vi "Close.vi"(8 "error in":errorcluster, 11 "Cycler in":refnum<class "Cycler.lvclass">) -> (0 "error out":errorcluster, 3 "Cycler out":refnum<class "Cycler.lvclass">)   [LabVIEW 2023, in "Cycler.lvclass"]
uses:
  Cycler.lvclass
  Cycler.lvclass/Cycler.ctl
  Low Level Capabilities/OnOff/OnOff.lvclass
  Low Level Capabilities/Output Enable/Output Enable.lvclass
  Low Level Capabilities/Control Mode/Control Mode.lvclass
  Low Level Capabilities/Current/Current Actual Value/Current Actual Value.lvclass
  Low Level Capabilities/Current/Current Gradient/Current Gradient.lvclass
  Low Level Capabilities/Current/Current Limit/Current Limit.lvclass
  Low Level Capabilities/Current/Current Setpoint/Current Setpoint.lvclass
  Low Level Capabilities/Power/Power Actual Value/Power Actual Value.lvclass
  Low Level Capabilities/Power/Power Gradient/Power Gradient.lvclass
  Low Level Capabilities/Power/Power Limit/Power Limit.lvclass
  Low Level Capabilities/Power/Power Setpoint/Power Setpoint.lvclass
  Low Level Capabilities/Voltage/Voltage Actual Value/Voltage Actual Value.lvclass
  Low Level Capabilities/Voltage/Voltage Gradient/Voltage Gradient.lvclass
  Low Level Capabilities/Voltage/Voltage Limit/Voltage Limit.lvclass
  Low Level Capabilities/Voltage/Voltage Setpoint/Voltage Setpoint.lvclass
  Low Level Capabilities/Error/Error.lvclass
  Low Level Capabilities/Error Channels/Error Channels.lvclass
  Low Level Capabilities/Iso Measurement/Iso Measurement.lvclass
  Low Level Capabilities/Parallel Mode/Parallel Mode.lvclass
  Low Level Capabilities/Parameter Set/Parameter Set.lvclass
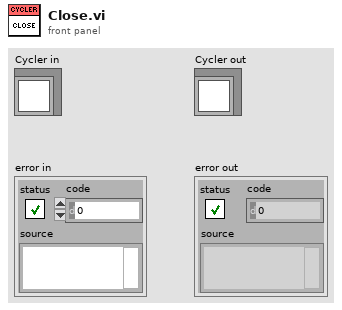
[diagram p1: front panel]
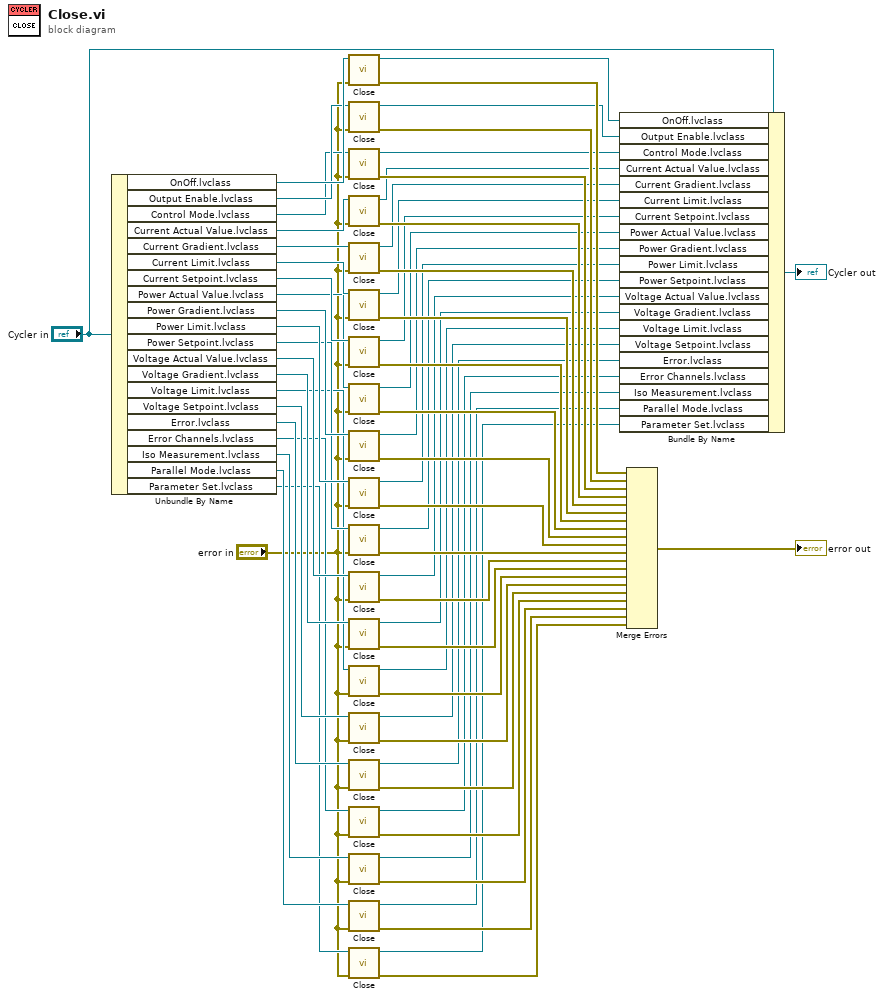
[diagram p0: block diagram]
diagram:
  n1 = Unbundle By Name("Cycler in") -> ("OnOff.lvclass"=w62:refnum<class "OnOff.lvclass">, "Output Enable.lvclass"=w59:refnum<class "Output Enable.lvclass">, "Control Mode.lvclass"=w56:refnum<class "Control Mode.lvclass">, "Current Actual Value.lvclass"=w53:refnum<class "Current Actual Value.lvclass">, "Current Gradient.lvclass"=w50:refnum<class "Current Gradient.lvclass">, "Current Limit.lvclass"=w47:refnum<class "Current Limit.lvclass">, "Current Setpoint.lvclass"=w44:refnum<class "Current Setpoint.lvclass">, "Power Actual Value.lvclass"=w41:refnum<class "Power Actual Value.lvclass">, "Power Gradient.lvclass"=w38:refnum<class "Power Gradient.lvclass">, "Power Limit.lvclass"=w35:refnum<class "Power Limit.lvclass">, "Power Setpoint.lvclass"=w32:refnum<class "Power Setpoint.lvclass">, "Voltage Actual Value.lvclass"=w29:refnum<class "Voltage Actual Value.lvclass">, "Voltage Gradient.lvclass"=w26:refnum<class "Voltage Gradient.lvclass">, "Voltage Limit.lvclass"=w23:refnum<class "Voltage Limit.lvclass">, "Voltage Setpoint.lvclass"=w20:refnum<class "Voltage Setpoint.lvclass">, "Error.lvclass"=w17:refnum<class "Error.lvclass">, "Error Channels.lvclass"=w14:refnum<class "Error Channels.lvclass">, "Iso Measurement.lvclass"=w11:refnum<class "Iso Measurement.lvclass">, "Parallel Mode.lvclass"=w6:refnum<class "Parallel Mode.lvclass">, "Parameter Set.lvclass"=w5:refnum<class "Parameter Set.lvclass">)
  n2 = call-dynamic "Close.vi"("error in"="error in", "OnOff in"=w62) -> ("error out"=w60:errorcluster, "OnOff out"=w61:refnum<class "OnOff.lvclass">)  [unwired: 8 in]
  n3 = call-dynamic "Close.vi"("error in"="error in", "Output Enable in"=w59) -> ("error out"=w57:errorcluster, "Output Enable out"=w58:refnum<class "Output Enable.lvclass">)  [unwired: 8 in]
  n4 = call-dynamic "Close.vi"("error in"="error in", "Control Mode in"=w56) -> ("error out"=w55:errorcluster, "Control Mode out"=w54:refnum<class "Control Mode.lvclass">)  [unwired: 8 in]
  n5 = call-dynamic "Close.vi"("error in"="error in", "Current Actual Value in"=w53) -> ("error out"=w52:errorcluster, "Current Actual Value out"=w51:refnum<class "Current Actual Value.lvclass">)  [unwired: 8 in]
  n6 = call-dynamic "Close.vi"("error in"="error in", "Current Gradient in"=w50) -> ("error out"=w49:errorcluster, "Current Gradient out"=w48:refnum<class "Current Gradient.lvclass">)  [unwired: 8 in]
  n7 = call-dynamic "Close.vi"("error in"="error in", "Current Limit in"=w47) -> ("error out"=w45:errorcluster, "Current Limit out"=w46:refnum<class "Current Limit.lvclass">)  [unwired: 8 in]
  n8 = call-dynamic "Close.vi"("error in"="error in", "Current Setpoint in"=w44) -> ("error out"=w43:errorcluster, "Current Setpoint out"=w42:refnum<class "Current Setpoint.lvclass">)  [unwired: 8 in]
  n9 = call-dynamic "Close.vi"("error in"="error in", "Power Actual Value in"=w41) -> ("error out"=w40:errorcluster, "Power Actual Value out"=w39:refnum<class "Power Actual Value.lvclass">)  [unwired: 8 in]
  n10 = call-dynamic "Close.vi"("error in"="error in", "Power Gradient in"=w38) -> ("error out"=w36:errorcluster, "Power Gradient out"=w37:refnum<class "Power Gradient.lvclass">)  [unwired: 8 in]
  n11 = call-dynamic "Close.vi"("error in"="error in", "Power Limit in"=w35) -> ("error out"=w34:errorcluster, "Power Limit out"=w33:refnum<class "Power Limit.lvclass">)  [unwired: 8 in]
  n12 = call-dynamic "Close.vi"("error in"="error in", "Power Setpoint in"=w32) -> ("error out"=w31:errorcluster, "Power Setpoint out"=w30:refnum<class "Power Setpoint.lvclass">)  [unwired: 8 in]
  n13 = call-dynamic "Close.vi"("error in"="error in", "Voltage Actual Value in"=w29) -> ("error out"=w27:errorcluster, "Voltage Actual Value out"=w28:refnum<class "Voltage Actual Value.lvclass">)  [unwired: 8 in]
  n14 = call-dynamic "Close.vi"("error in"="error in", "Voltage Gradient in"=w26) -> ("error out"=w24:errorcluster, "Voltage Gradient out"=w25:refnum<class "Voltage Gradient.lvclass">)  [unwired: 8 in]
  n15 = call-dynamic "Close.vi"("error in"="error in", "Voltage Limit in"=w23) -> ("error out"=w22:errorcluster, "Voltage Limit out"=w21:refnum<class "Voltage Limit.lvclass">)  [unwired: 8 in]
  n16 = call-dynamic "Close.vi"("error in"="error in", "Voltage Setpoint in"=w20) -> ("error out"=w18:errorcluster, "Voltage Setpoint out"=w19:refnum<class "Voltage Setpoint.lvclass">)  [unwired: 8 in]
  n17 = call-dynamic "Close.vi"("error in"="error in", "Error in"=w17) -> ("error out"=w15:errorcluster, "Error out"=w16:refnum<class "Error.lvclass">)  [unwired: 8 in]
  n18 = call-dynamic "Close.vi"("error in"="error in", "Error Channels in"=w14) -> ("error out"=w13:errorcluster, "Error Channels out"=w12:refnum<class "Error Channels.lvclass">)  [unwired: 8 in]
  n19 = call-dynamic "Close.vi"("error in"="error in", "Iso Measurement in"=w11) -> ("error out"=w9:errorcluster, "Iso Measurement out"=w10:refnum<class "Iso Measurement.lvclass">)  [unwired: 8 in]
  n20 = call-dynamic "Close.vi"("error in"="error in", "Parallel Mode in"=w6) -> ("error out"=w8:errorcluster, "Parallel Mode out"=w7:refnum<class "Parallel Mode.lvclass">)  [unwired: 8 in]
  n21 = call-dynamic "Close.vi"("error in"="error in", "Parameter Set in"=w5) -> ("error out"=w3:errorcluster, "Parameter Set out"=w4:refnum<class "Parameter Set.lvclass">)  [unwired: 8 in]
  n22 = Bundle By Name(cluster="Cycler in", "OnOff.lvclass"=w61, "Output Enable.lvclass"=w58, "Control Mode.lvclass"=w54, "Current Actual Value.lvclass"=w51, "Current Gradient.lvclass"=w48, "Current Limit.lvclass"=w46, "Current Setpoint.lvclass"=w42, "Power Actual Value.lvclass"=w39, "Power Gradient.lvclass"=w37, "Power Limit.lvclass"=w33, "Power Setpoint.lvclass"=w30, "Voltage Actual Value.lvclass"=w28, "Voltage Gradient.lvclass"=w25, "Voltage Limit.lvclass"=w21, "Voltage Setpoint.lvclass"=w19, "Error.lvclass"=w16, "Error Channels.lvclass"=w12, "Iso Measurement.lvclass"=w10, "Parallel Mode.lvclass"=w7, "Parameter Set.lvclass"=w4) -> (→"Cycler out":refnum<class "Cycler.lvclass">)
  n23 = Merge Errors(w60, w57, w55, w52, w49, w45, w43, w40, w36, w34, w31, w27, w24, w22, w18, w15, w13, w9, w8, w3) -> (→"error out":errorcluster)
